vi "TransverseSensing.vi"(10 "SensorInputData":T5, 11 "HMI to Control":T1) -> (2 "SensorInputDataOut":T5, 3 "HMI to ControlOut":T1, 4 "Done":bool=TRUE)   [LabVIEW 2015]
uses:
  Typedefs/SensorInputData.ctl
  Typedefs/HMI_to_Control.ctl
  Typedefs/Arm States.ctl
  Typedefs/ClawStates.ctl
  Typedefs/IntakeWheelSenseOrManual.ctl
panel:
  in  "arguments":string[](array[string])
  in  "dt":i32
  in  "Reinit":bool
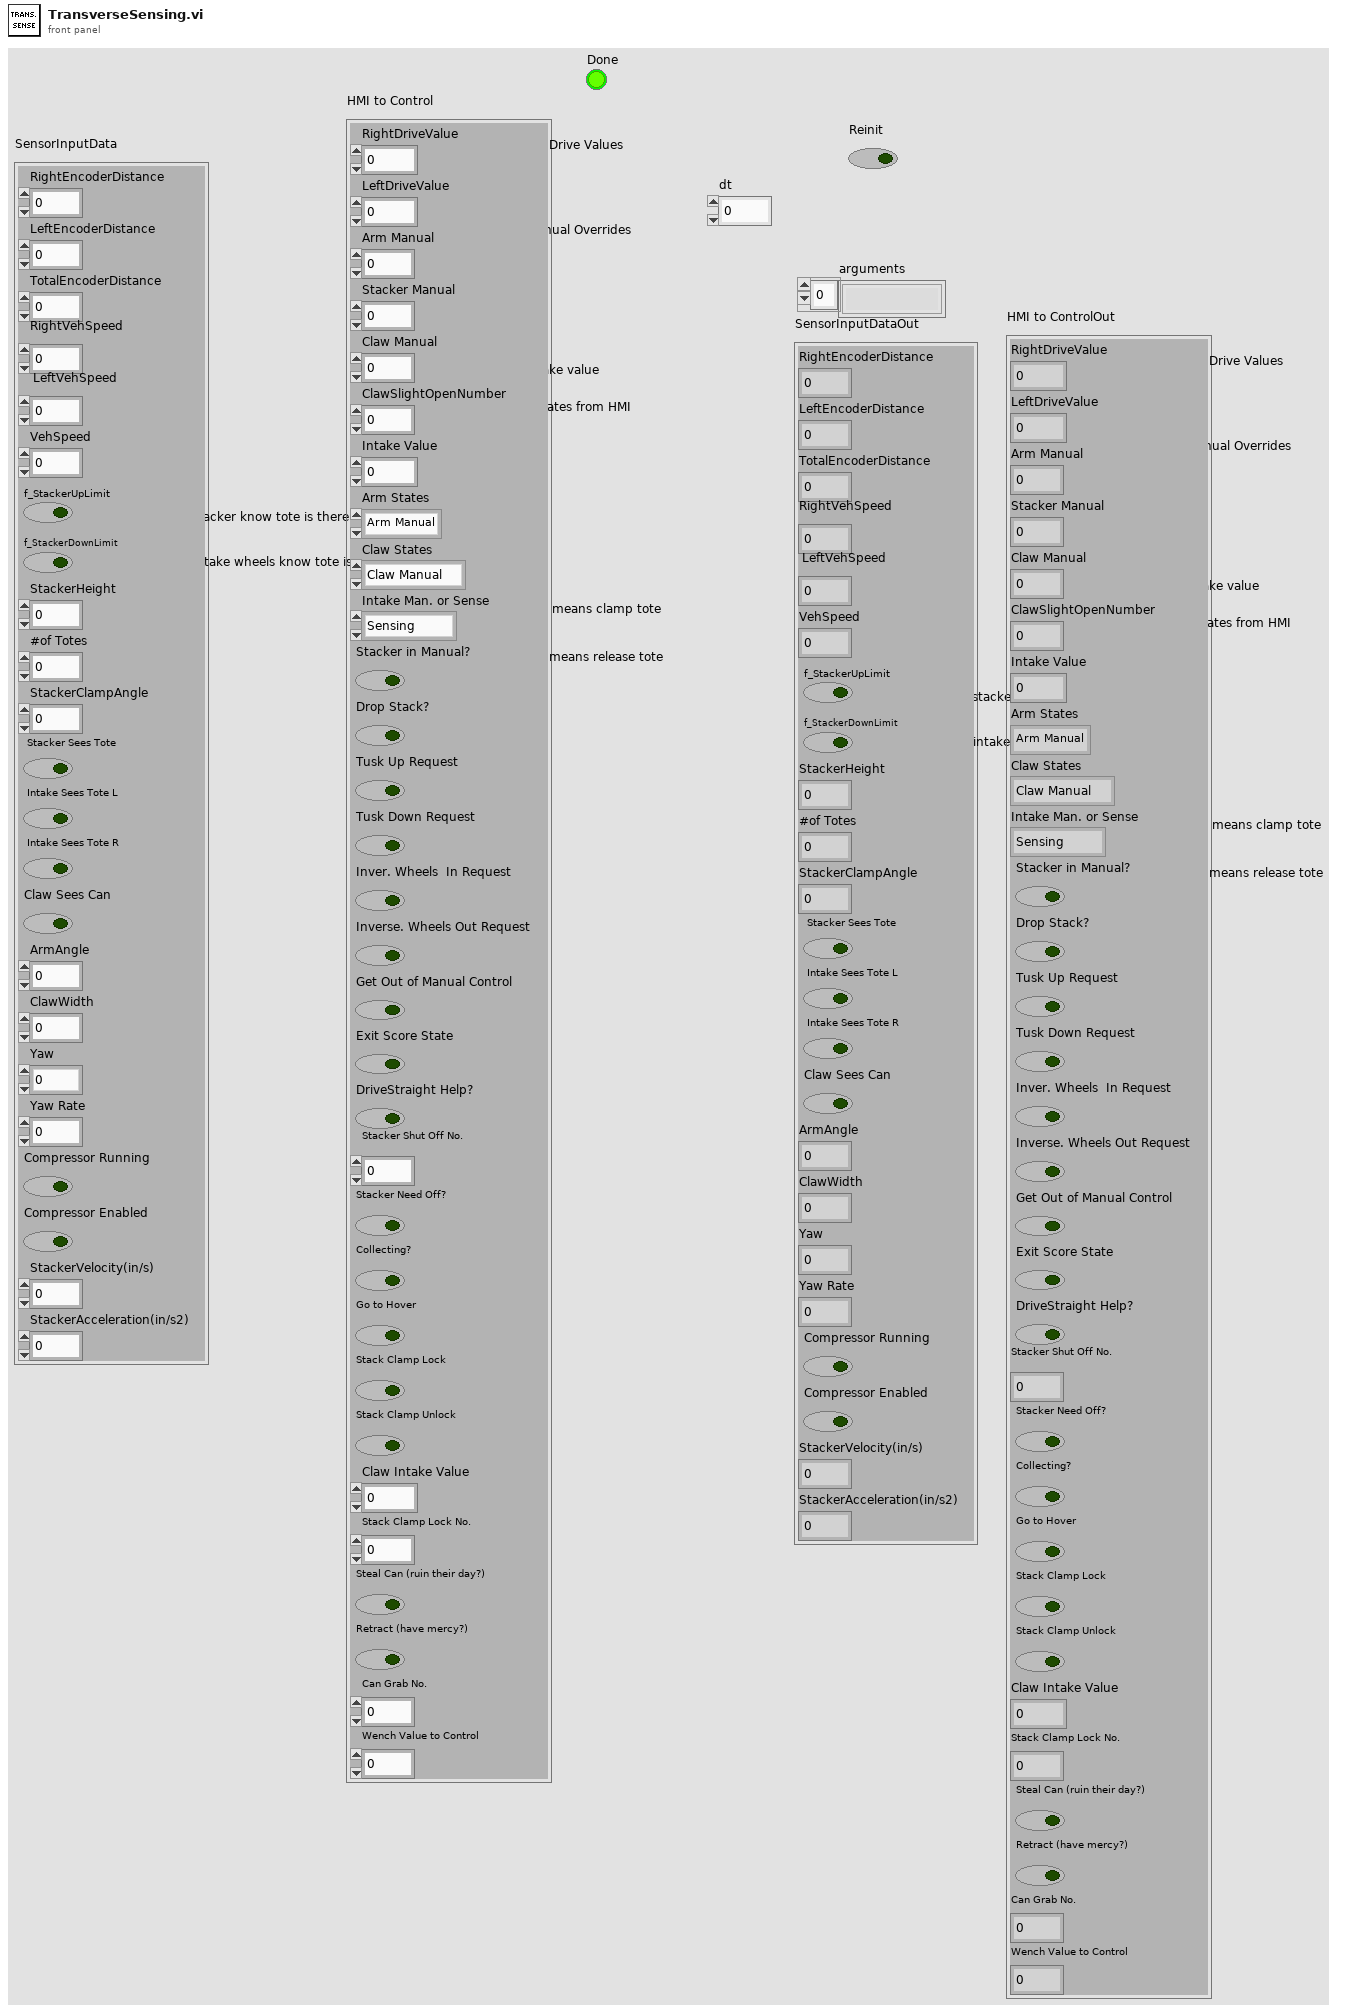
[diagram p1: front panel]
types:
  T1 = typedef "HMI_to_Control.ctl" = cluster{"RightDriveValue":dbl, "LeftDriveValue":dbl, "Arm Manual ":dbl, "Stacker Manual ":dbl, "Claw Manual ":dbl, "ClawSlightOpenNumber":i8, "Intake Value ":sgl, "Arm States":T2, "Claw States":T3, "Intake Man. or Sense":T4, "Stacker in Manual?":bool, "Drop Stack? ":bool, "Tusk Up Request":bool, "Tusk Down Request":bool, "Inver. Wheels  In Request":bool, "Inverse. Wheels Out Request ":bool, "Get Out of Manual Control":bool, "Exit Score State":bool, "DriveStraight Help?":bool, "Stacker Shut Off No.":i8, "Stacker Need Off?":bool, "Collecting?":bool, "Go to Hover":bool, "Stack Clamp Lock ":bool, "Stack Clamp Unlock ":bool, "Claw Intake Value ":sgl, "Stack Clamp Lock No. ":i8, "Steal Can (ruin their day?)":bool, "Retract (have mercy?)":bool, "Can Grab No. ":i8, "Wench Value to Control ":dbl}
  T2 = typedef "Arm States.ctl" = enum16{"Arm Manual ", "Ground", "Step", "1 Tote", "2 Tote", "3 Tote", "4 Tote", "5 Tote", "6 Tote", "Flip Can Arm", "Grab Can in auto", "Nudge"}
  T3 = typedef "ClawStates.ctl" = enum16{"Claw Manual ", "Claw Open", "Claw Closed", "Claw Slight Open", "Flip Can"}
  T4 = typedef "IntakeWheelSenseOrManual.ctl" = enum16{"Sensing", "Manual "}
  T5 = typedef "SensorInputData.ctl" = cluster{"RightEncoderDistance":dbl, "LeftEncoderDistance":dbl, "TotalEncoderDistance":dbl, "RightVehSpeed":dbl, "LeftVehSpeed":dbl, "VehSpeed":dbl, "f_StackerUpLimit":bool, "f_StackerDownLimit":bool, "StackerHeight":dbl, "#of Totes":u8, "StackerClampAngle":dbl, "Stacker Sees Tote":bool, "Intake Sees Tote L":bool, "Intake Sees Tote R":bool, "Claw Sees Can":bool, "ArmAngle":dbl, "ClawWidth":dbl, "Yaw":dbl, "Yaw Rate":dbl, "Compressor Running":bool, "Compressor Enabled":bool, "StackerVelocity(in/s)":dbl, "StackerAcceleration(in/s2)":dbl}
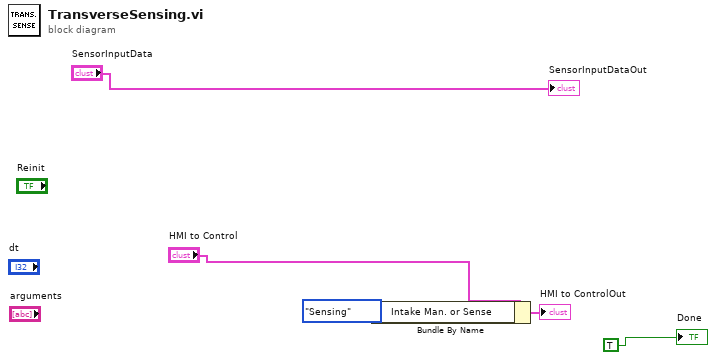
[diagram p0: block diagram]
diagram:
  n1 = Bundle By Name(cluster="HMI to Control", "Intake Man. or Sense"=IntakeWheelSenseOrManual."Sensing") -> (→"HMI to ControlOut":T1)
  "SensorInputDataOut" <- "SensorInputData"
  "Done" <- TRUE
